vi "Time series save images.vi"(7 "Logging queue":refnum<queue>, 8 "error in (no error)":errorcluster, 9 "Ch1-Green":i16[][](array[numeric]), 10 "Ch0-Red":i16[][](array[numeric]), 11 "Logging queue element":T1={"Imaging Protocol"=enum."Live Imaging", "Number of Trials"=0, "Frame Size"=512, "# Averaged frames"=0, "Dwell time (us)"=0.0, "Index of Z-plane"=0, "Timelapse?"=FALSE, "Logging process is active"=FALSE, "Speed logging enabled"=FALSE, "tdms file ref"=refnum, "path"=path "", "Trial Number"=0, "Expected # points acquired"=FALSE, "Manually stopped"=FALSE, "Last trial"=FALSE, "Ch0 data"=[], "Ch1 data"=[], "Ref Data"=[], "Ref Frame Time"=[], "Image Time"=[], "Continuous Time"=[], "Ref X Length"=0, "Ref Y Length"=0, "# Ref Averaged frames"=0, "Ref Dwell time (us)"=0.0, "Points acquired"={"Ch0 last trial"=0, "Ch1 last trial"=0, "All trials"=0}, "HW Timings File"=refnum} {"Ref Dwell time (us)" format="%#.6g"; "Frame Size" items=["100X100"=100, "128X128"=128, "200X200"=200, "256X256"=256, "512X512"=512, "1024x1024"=1024, "2048x2048"=2048]; "Dwell time (us)" format="%#.6g"}) -> (0 "error":errorcluster)   [LabVIEW 2020]
uses:
  Typedefs/Logging queue element.ctl
  Typedefs/Imaging Protocols enum.ctl
  Typedefs/Frame Size.ctl
  Typedefs/Acquired points count.ctl
  Typedefs/Read Write Enum.ctl
  Typedefs/Channel Selector.ctl
  Typedefs/Top level VI states.ctl
  Global Variables/General Globals.vi
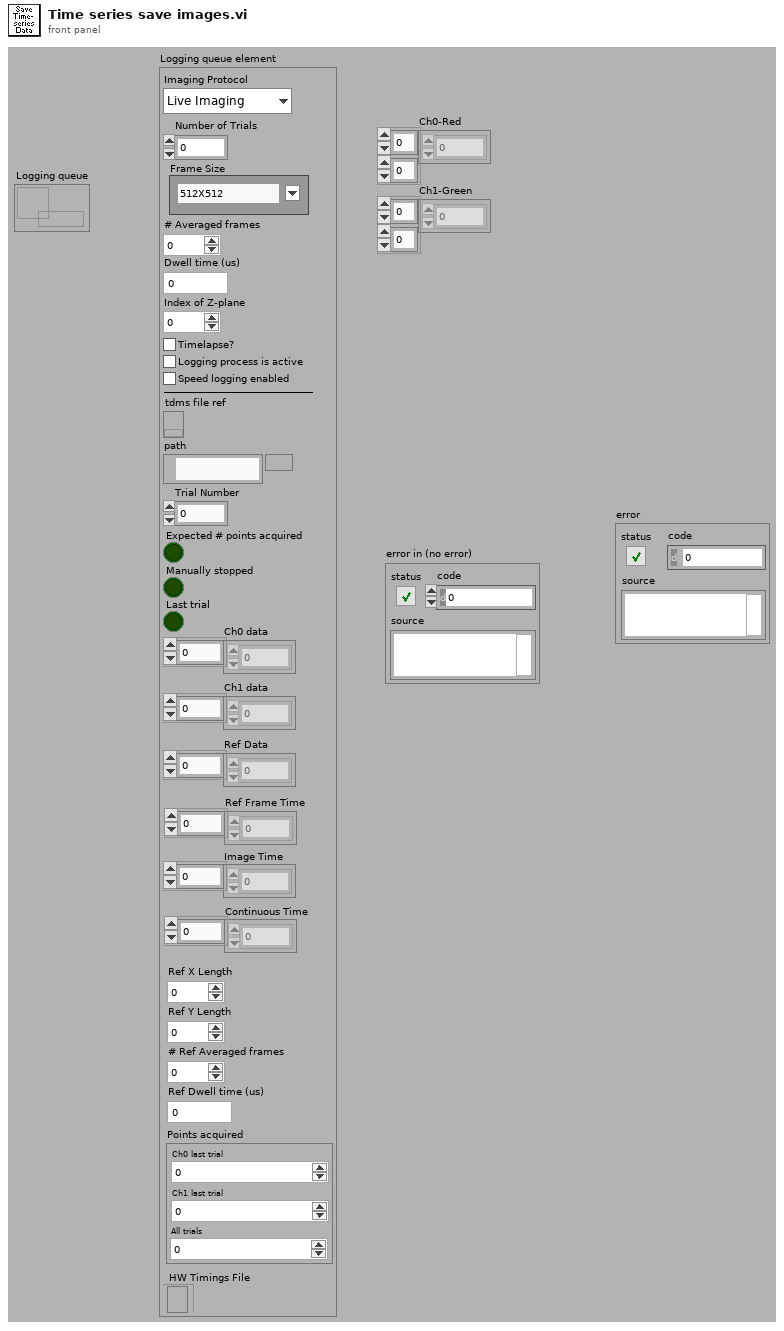
[diagram p1: front panel]
types:
  T1 = typedef "Logging queue element.ctl" = cluster{"Imaging Protocol":T2, "Number of Trials":u16, "Frame Size":T3, "# Averaged frames":u16, "Dwell time (us)":dbl, "Index of Z-plane":i32, "Timelapse?":bool, "Logging process is active":bool, "Speed logging enabled":bool, "tdms file ref":refnum<k34>, "path":path, "Trial Number":i32, "Expected # points acquired":bool, "Manually stopped":bool, "Last trial":bool, "Ch0 data":u32[], "Ch1 data":u32[], "Ref Data":u32[], "Ref Frame Time":u64[], "Image Time":u64[], "Continuous Time":u64[], "Ref X Length":u16, "Ref Y Length":u16, "# Ref Averaged frames":u16, "Ref Dwell time (us)":dbl, "Points acquired":T4, "HW Timings File":refnum<file>}
  T2 = typedef "Imaging Protocols enum.ctl" = enum16{"AOL Z-Stack", "Motor Z Stack", "Functional Acquisition", "Single Plane Acquisition", "Volume Acquisition", "Live Imaging", "Live Plane Imaging", "Live Volume Imaging"}
  T3 = typedef "Frame Size.ctl" = u16
  T4 = typedef "Acquired points count.ctl" = cluster{"Ch0 last trial":u64, "Ch1 last trial":u64, "All trials":u64}
  T5 = typedef "Read Write Enum.ctl" = enum16{"Read", "Write"}
  T6 = typedef "Channel Selector.ctl" = enum16{"Red Channel", "Green Channel", "Blended"}
  T7 = typedef "Top level VI states.ctl" = enum16{"None", "Initialise UI", "<STACK PROTOCOL STATES>", "AOL Zstack-START", "AOL Zstack-STOP", "Motor Zstack-START", "Motor Zstack-STOP", "<ACQUISITION PROTOCOL STATES> ", "Functional Acquisition-START", "Functional Acquisition-STOP", "Single Plane Acquisition-START", "Single Plane Acquisition-STOP", "Volume Acquisition-START", "Volume Acquisition-STOP", "<LIVE IMAGING PROTOCOL STATES>", "Live Imaging-START", "Live Imaging-STOP", "Live Plane Imaging-START", "Live Plane Imaging-STOP", "Live Volume Imaging-START", "Live Volume Imaging-STOP", "<MOVEMENT CORRECTION PROTOCOL STATES>", "EXIT"}
  T8 = typedef "AVI implementation enum.ctl" = enum16{"AVI1", "AVI2"}
  T9 = typedef "AVI Refs cluster.ctl" = cluster{"AVI2 path":path, "AVI 2 Refnum":T10, "New Image":T11, "error out":errorcluster, "Avi 1 Refnum":T12}
  T10 = typedef "IMAQ AVI2 Refnum.ctl" = refnum<k20>
  T11 = typedef "IMAQ Image.ctl" = refnum<image>
  T12 = typedef "AviRefnum.ctl" = refnum<k1>
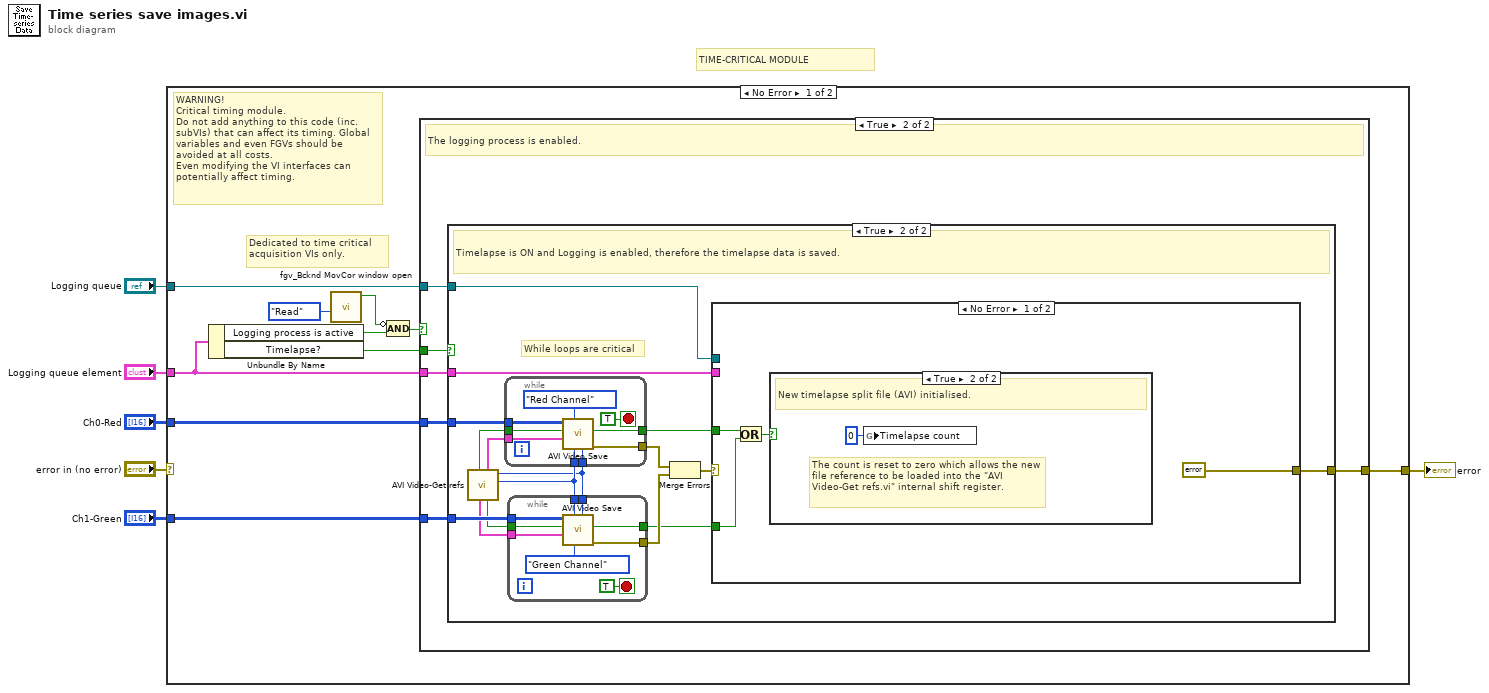
[diagram p0: block diagram]
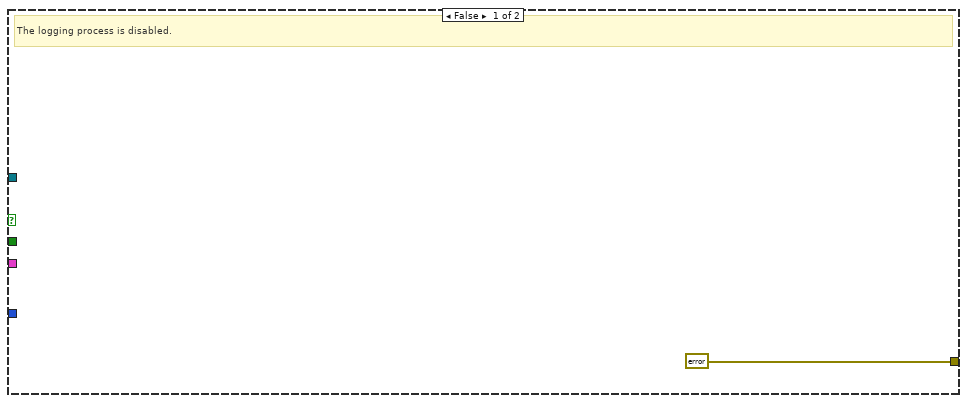
[diagram p2: hidden frame]
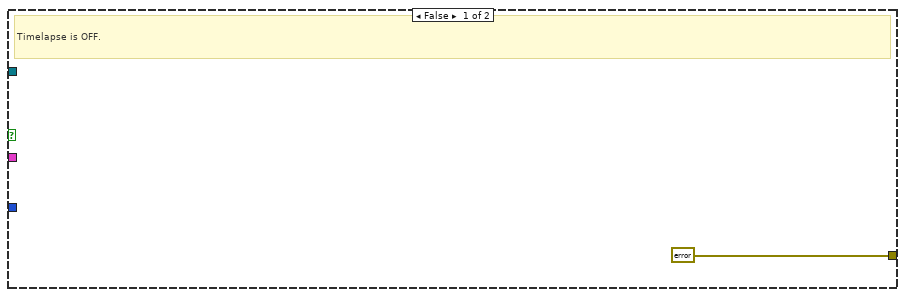
[diagram p3: hidden frame]
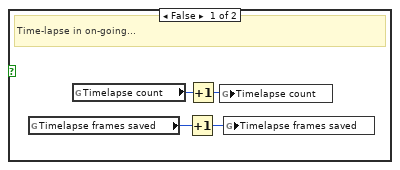
[diagram p4: hidden frame]
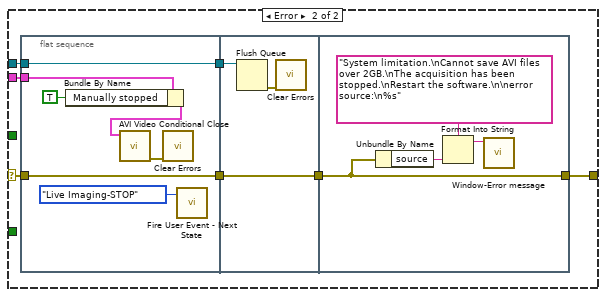
[diagram p5: hidden frame]
diagram:
  # "TIME-CRITICAL MODULE"
  n1 = case shown="No Error" "error in (no error)" {
    selector: "error in (no error)" -> [_ w89]
    tunnel: [w16 w89] -> w6
    tunnel: "Logging queue element" -> [w9 _]
    tunnel: "Ch0-Red" -> [w15 _]
    tunnel: "Ch1-Green" -> [w14 _]
    tunnel: "Logging queue" -> [w12 _]
    frame No Error {
      # "WARNING!\nCritical timing module.\nDo not add anything to this code (inc. subVIs) that can affect its timing. Global variables and even FGVs should be avoided at all costs.\nEven modifying the VI interfaces can potentially affect timing."
      # "Dedicated to time critical acquisition VIs only."
      n2 = Unbundle By Name(w9) -> ("Logging process is active"=w11:bool, "Timelapse?"=w13:bool)
      n3 = call "fgv_Bcknd MovCor window open.vi"("Function"=Read_Write_Enum."Read") -> ("Background MovCor window is open"=w7:bool)  [unwired: 9 in, 1 out]
      n4 = Compound Arithmetic op=AND(invert w7, w11) -> (w10:bool)
      n5 = case shown="True" w10 {
        tunnel: [errorcluster {"status"=FALSE, "code"=0, "source"=""} ("error IO") w23] -> w16
        tunnel: w15 -> [_ w22]
        tunnel: w14 -> [_ w21]
        tunnel: w13 -> [_ w20]
        tunnel: w9 -> [_ w19]
        tunnel: w12 -> [_ w18]
        frame False {
          # "The logging process is disabled."
        }
        frame True {
          # "The logging process is enabled."
          n6 = case shown="True" w20 {
            tunnel: [errorcluster {"status"=FALSE, "code"=0, "source"=""} ("error IO") w29] -> w23
            tunnel: w22 -> [_ w38]
            tunnel: w21 -> [_ w37]
            tunnel: w19 -> [_ w31]
            tunnel: w18 -> [_ w30]
            frame False {
              # "Timelapse is OFF."
            }
            frame True {
              # "While loops are critical"
              # "Timelapse is ON and Logging is enabled, therefore the timelapse data is saved."
              n7 = call "AVI Video-Get refs.vi"() -> ("AVI mode"=w32:T8, "Frame Size"=w25:u32, "Green PMT is ON"=w34:bool, "Red AVI"=w35:T9, "Green AVI"=w33:T9, "Red PMT is ON"=w36:bool)  [unwired: 5 in, 1 out]
              n8 = while {
                tunnel: [w58] -> w39
                tunnel: w38 -> [w57]
                tunnel: w36 -> [w56]
                tunnel: w35 -> [w55]
                tunnel: w32 -> [w54]
                tunnel: [w52] -> w26
                tunnel: w25 -> [w51]
                stop <- TRUE stop-if-true
                n9 = call "AVI Video Save.vi"("Frame Size"=w51, "Channel"=Channel_Selector."Red Channel", "AVI mode"=w54, "AVI cluster"=w55, "PMT is ON?"=w56, "Image Pixels"=w57) -> ("error out"=w58:errorcluster, "New split file has just been initialised"=w52:bool)  [unwired: 4 in]
              }
              n10 = while {
                tunnel: [w49] -> w40
                tunnel: w37 -> [w48]
                tunnel: w34 -> [w47]
                tunnel: w33 -> [w46]
                tunnel: w32 -> [w45]
                tunnel: [w43] -> w27
                tunnel: w25 -> [w42]
                stop <- TRUE stop-if-true
                n11 = call "AVI Video Save.vi"("Frame Size"=w42, "Channel"=Channel_Selector."Green Channel", "AVI mode"=w45, "AVI cluster"=w46, "PMT is ON?"=w47, "Image Pixels"=w48) -> ("error out"=w49:errorcluster, "New split file has just been initialised"=w43:bool)  [unwired: 4 in]
              }
              n12 = Merge Errors(w39, w40) -> (w28:errorcluster)
              n13 = case shown="No Error" w28 {
                selector: w28 -> [_ w69]
                tunnel: w31 -> [_ w74]
                tunnel: w30 -> [_ w73]
                tunnel: [errorcluster {"status"=FALSE, "code"=0, "source"=""} ("error IO") w68] -> w29
                tunnel: w27 -> [w61 _]
                tunnel: w26 -> [w62 _]
                frame No Error {
                  n14 = Or(x=w62, y=w61) -> (x .or. y?=w60:bool)
                  n15 = case shown="True" w60 {
                    frame False {
                      # "Time-lapse in on-going..."
                      n16 = global read "General Globals.vi" "Timelapse frames saved"() -> (w64:u32)
                      n17 = global read "General Globals.vi" "Timelapse count"() -> (w65:u32)
                      n18 = Increment(x=w64) -> (x+1=w63:u32)
                      n19 = Increment(x=w65) -> (x+1=w66:u32)
                      n20 = global write "General Globals.vi" "Timelapse count"(w66) -> ()
                      n21 = global write "General Globals.vi" "Timelapse frames saved"(w63) -> ()
                    }
                    frame True {
                      # "The count is reset to zero which allows the new file reference to be loaded into the \"AVI Video-Get refs.vi\" internal shift register."
                      # "New timelapse split file (AVI) initialised."
                      n22 = global write "General Globals.vi" "Timelapse count"(u32 0 ("Timelapse count")) -> ()
                    }
                  }
                }
                frame Error {
                  n23 = flat-sequence {
                    tunnel: w74 -> [w80]
                    tunnel: [w77] -> w72
                    tunnel: w73 -> [w77]
                    tunnel: [w75] -> w70
                    tunnel: w69 -> [w75]
                    tunnel: w72 -> [w83]
                    tunnel: [w82] -> w71
                    tunnel: w70 -> [w82]
                    tunnel: w71 -> [w85]
                    tunnel: [w85] -> w68
                    frame #0 {
                      n24 = Bundle By Name(cluster=w80, "Manually stopped"=TRUE) -> (w78:T1)
                      n25 = call "AVI Video Conditional Close.vi"("Logging queue element in"=w78) -> ("error out"=w81:errorcluster)  [unwired: 10 in]
                      n26 = call <vilib>:"Clear Errors.vi"("error in (no error)"=w81) -> ()  [unwired: 5 in, 2 out]
                      n27 = call "Fire User Event - Next State.vi"("\"UI Handler loop\" case to execute"=Top_level_VI_states."Live Imaging-STOP" ("event data / imaging mode")) -> ()  [unwired: 10 in, 1 out]
                    }
                    frame #1 {
                      n28 = Flush Queue(queue=w83) -> (error out=w84:errorcluster)  [unwired: 1 in, 2 out]
                      n29 = call <vilib>:"Clear Errors.vi"("error in (no error)"=w84) -> ()  [unwired: 5 in, 2 out]
                    }
                    frame #2 {
                      n30 = Unbundle By Name(w85) -> ("source"=w87:string)
                      n31 = Format Into String(format string="System limitation.\nCannot save AVI files over 2GB.\nThe acquisition has been stopped.\nRestart the software.\n\nerror source:\n%s", w87) -> (resulting string=w86:string)  [unwired: 2 in, 1 out]
                      n32 = call "Window-Error message.vi"("Message"=w86) -> ()  [unwired: 10 in, 1 out]
                    }
                  }
                }
              }
            }
          }
        }
      }
    }
    frame Error {
    }
  }
  "error" <- w6
